vi "Proyecto Control A.vi"() -> ()   [LabVIEW 2015]
uses:
  <vilib>/Instr/_visa.llb/VISA Configure Serial Port (Instr).vi
panel:
  in  "Boolean":bool
  in  "Man / Aut":bool
  in  "stop":bool
  out "substring":string
  out "String":string
  out "Distancia":u8
  in  "VISA resource name":refnum<visa-resource-name>
  out "read buffer":string
  out "Waveform Chart":cluster{"Set Point":u8, u8}(graph)
  in  "Set Point":u8
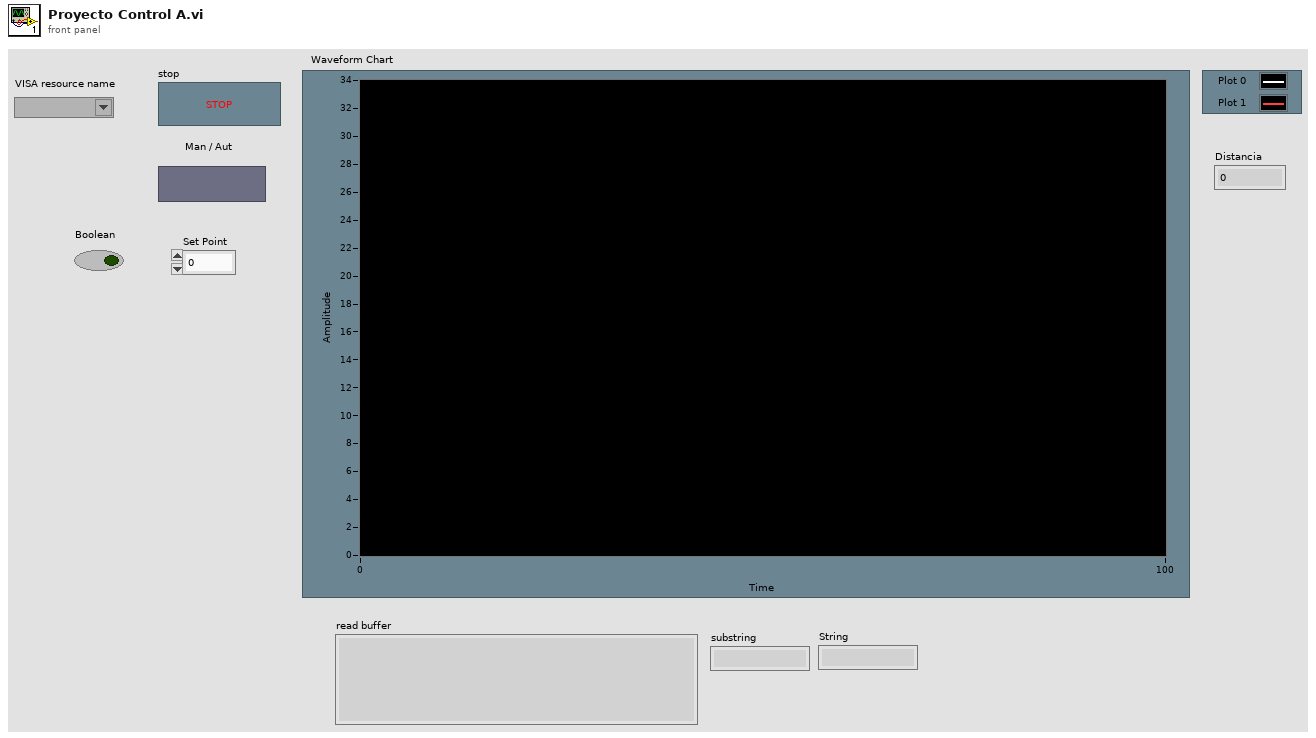
[diagram p1: front panel]
types:
  T1 = enum16{"open", "replace", "create", "open or create", "replace or create", "replace or create with confirmation"}
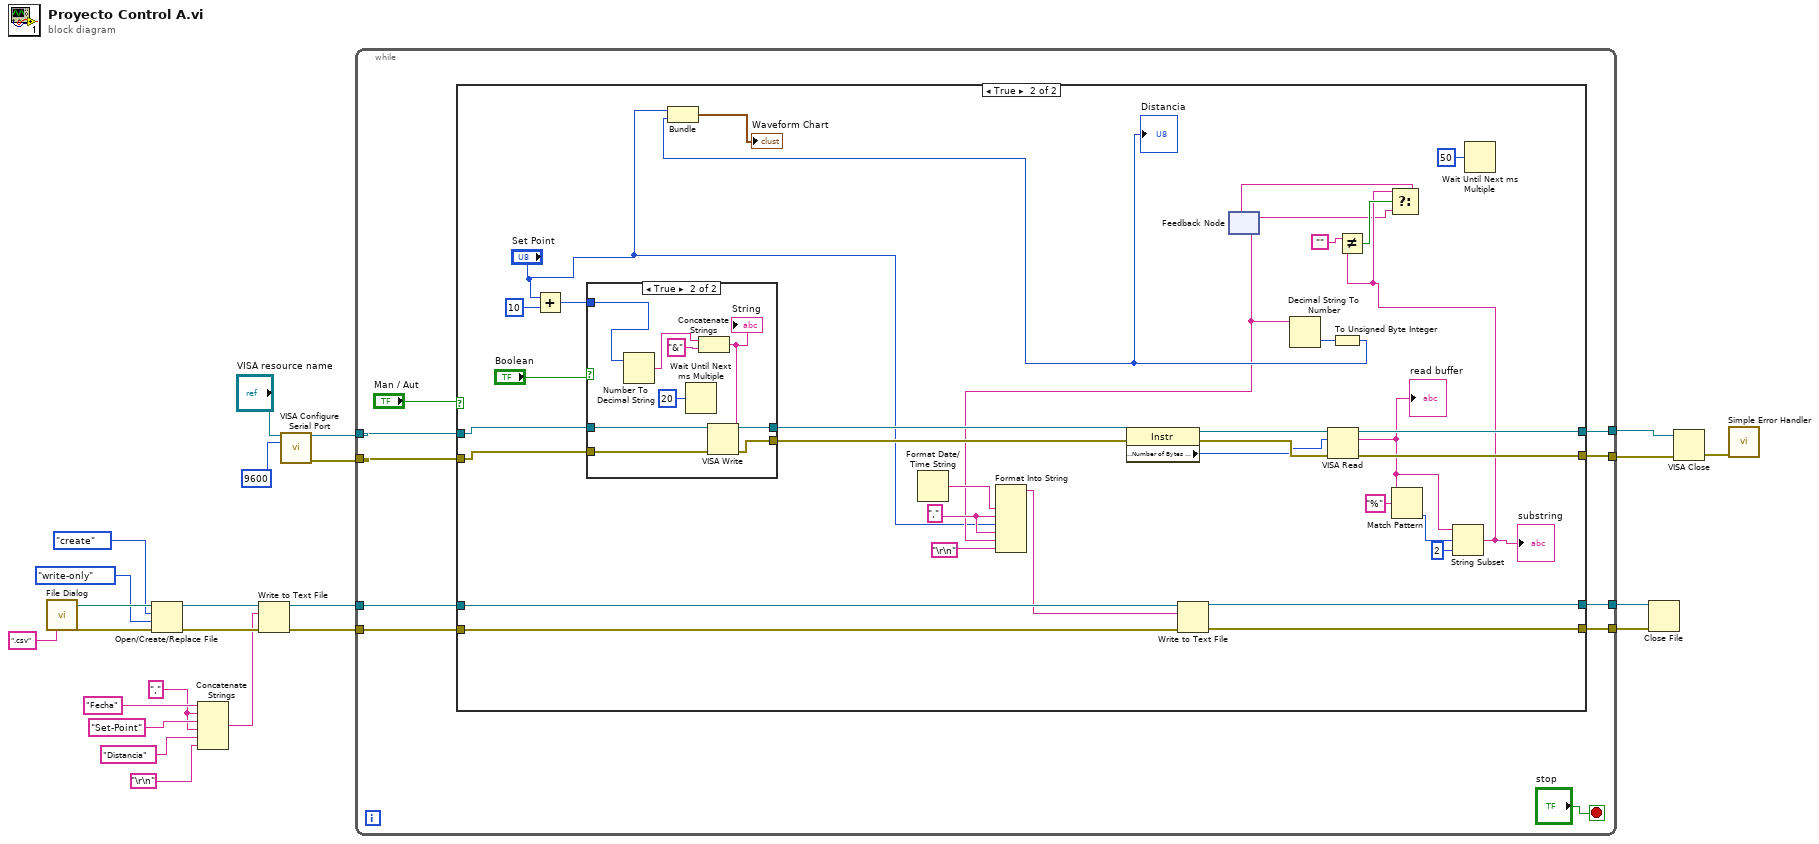
[diagram p0: block diagram]
diagram:
  w9 = ","
  n1 = call "File Dialog"("pattern (all files)"=".csv") -> ("selected path"=w15:path, "error out"=w14:errorcluster)  [unwired: 11 in, 2 out]
  n2 = Open/Create/Replace File(file path (use dialog)=w15, error in=w14, operation (0:open)=T1."create", access (0:read/write)=enum16{"read/write", "read-only", "write-only"}."write-only") -> (refnum out=w4:refnum<file>, error out=w3:errorcluster)  [unwired: 2 in, 1 out]
  n3 = Concatenate Strings("Fecha" ("string"), w9, "Set-Point" ("string"), w9, "Distancia" ("string"), "\r\n") -> (w2:string)
  n4 = Write to Text File(file (use dialog)=w4, text=w2, error in=w3) -> (refnum out=w6:refnum<file>, error out=w5:errorcluster)  [unwired: 1 in, 1 out]
  n5 = call-poly "VISA Configure Serial Port"("VISA resource name"="VISA resource name", "baud rate (9600)"=u32 9600) -> ("VISA resource name out"=w24:refnum<visa-resource-name>, "error out"=w23:errorcluster)  [unwired: 12 in]
  n6 = while {
    tunnel: w24 -> [w34]
    tunnel: w23 -> [w33]
    tunnel: [w32] -> w22
    tunnel: [w31] -> w21
    tunnel: w6 -> [w28]
    tunnel: w5 -> [w27]
    tunnel: [w26] -> w18
    tunnel: [w25] -> w17
    stop <- "stop" stop-if-true
    n7 = case shown="True" "Man / Aut" {
      tunnel: w34 -> [w38 w72]
      tunnel: w33 -> [w37 w71]
      tunnel: [w38 w70] -> w32
      tunnel: [w37 w69] -> w31
      tunnel: w28 -> [w36 w44]
      tunnel: w27 -> [w35 w43]
      tunnel: [w36 w41] -> w26
      tunnel: [w35 w40] -> w25
      frame False {
      }
      frame True {
        w47 = ","
        n8 = Add(x="Set Point", y=u8 10) -> (x+y=w50:u8)
        n9 = case shown="True" "Boolean" {
          tunnel: w72 -> [w74 w83]
          tunnel: w71 -> [w73 w82]
          tunnel: [w74 w79] -> w58
          tunnel: [w73 w78] -> w57
          tunnel: w50 -> [_ w77]
          frame False {
          }
          frame True {
            n10 = Number To Decimal String(number=w77) -> (decimal integer string=w80:string)  [unwired: 1 in]
            n11 = Wait Until Next ms Multiple(millisecond multiple=u32 20) -> ()  [unwired: 1 out]
            n12 = Concatenate Strings(w80, "&" ("string")) -> (w76:string)
            "String" <- w76
            n13 = VISA Write(VISA resource name=w83, write buffer=w76, error in (no error)=w82) -> (VISA resource name out=w79:refnum<visa-resource-name>, error out=w78:errorcluster)  [unwired: 1 out]
          }
        }
        n14 = Format Date/Time String() -> (date/time string=w49:string)  [unwired: 3 in]
        n15 = property class="Instr"(reference=w58, error in=w57) -> (reference out=w68:refnum<visa-resource-name>, error out=w67:errorcluster, "Serial Settings:Number of Bytes at Serial Port"=w55:u32)
        n16 = feedback #1() -> (w46:string)  [unwired: 1 in]
        n17 = Format Into String(w49, w47, "Set Point", w47, w46, "\r\n") -> (resulting string=w42:string)  [unwired: 3 in, 1 out]
        n18 = Write to Text File(file (use dialog)=w44, text=w42, error in=w43) -> (refnum out=w41:refnum<file>, error out=w40:errorcluster)  [unwired: 1 in, 1 out]
        n19 = Decimal String To Number(string=w46) -> (number=w65:i32)  [unwired: 2 in, 1 out]
        n20 = VISA Read(VISA resource name=w68, byte count=w55, error in (no error)=w67) -> (VISA resource name out=w70:refnum<visa-resource-name>, read buffer=w53:string, error out=w69:errorcluster)  [unwired: 1 out]
        "read buffer" <- w53
        n21 = To Unsigned Byte Integer(number=w65) -> (unsigned 8bit integer=w48:u8)
        "Distancia" <- w48
        n22 = Bundle("Set Point"="Set Point", w48) -> (→"Waveform Chart":cluster{"Set Point":u8, u8})  [unwired: 1 in]
        n23 = Match Pattern(string=w53, regular expression="%") -> (offset past match=w52:i32)  [unwired: 1 in, 3 out]
        n24 = String Subset(string=w53, offset (0)=w52, length (rest)=2 ("length (rest)")) -> (substring=w60:string)
        "substring" <- w60
        n25 = Not Equal?(x="", y=w60) -> (x != y?=w63:bool)
        n26 = Select(t=w60, s=w63, f=w46) -> (s? t:f=w62:string)
        n27 = feedback-in #1(w62) -> ()
        n28 = Wait Until Next ms Multiple(millisecond multiple=u32 50) -> ()  [unwired: 1 out]
      }
    }
  }
  n29 = Close File(refnum=w18, error in=w17) -> ()  [unwired: 2 out]
  n30 = VISA Close(VISA resource name=w22, error in (no error)=w21) -> (error out=w1:errorcluster)
  n31 = call <vilib>:"Simple Error Handler.vi"("error in (no error)"=w1) -> ()  [unwired: 4 in, 5 out]
